vi "G#Template_CreateSub.vi"(0 "reference in":refnum<class "G#Template.lvclass">, 5 "error in (no error)":errorcluster) -> (14 "reference out":refnum<class "G#Template.lvclass">, 19 "error out":errorcluster)   [LabVIEW 2020, in "G#Template.lvclass"]
doc: "Constructor."
uses:
  G#Template.lvclass
  C:/ProjectGSharpDevelopment_2020-3/gsharp/VIPM/Files/vi.lib/addons/_AddQ/G#Object/G#Object.lvclass
  G#Object/G#Object.lvclass
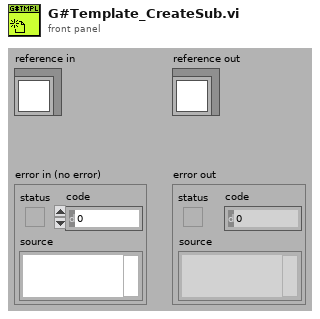
[diagram p1: front panel]
types:
  T1 = typedef "G#Template.lvclass/ObjectAttributesRef.ctl" = refnum<data-value>
  T2 = typedef "G#Template.lvclass/ObjectAttributes.ctl" = cluster{"MyAttribute":dbl}
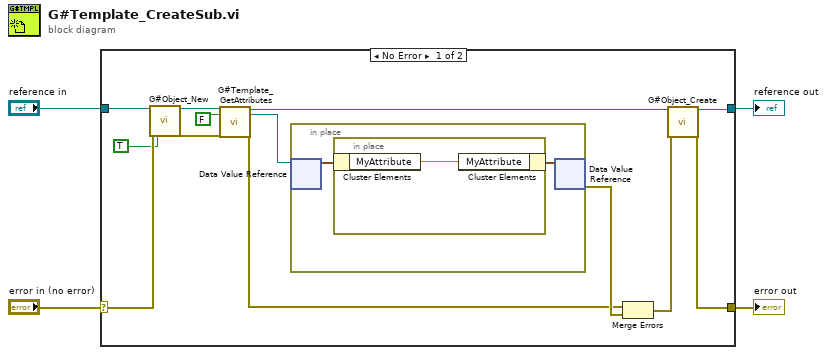
[diagram p0: block diagram]
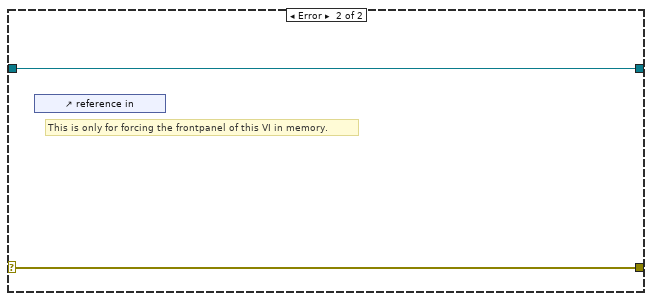
[diagram p2: hidden frame]
diagram:
  n1 = case shown="No Error" "error in (no error)" {
    selector: "error in (no error)" -> [w16 w22]
    tunnel: [w6 w22] -> w3
    tunnel: [w8 w21] -> w1
    tunnel: "reference in" -> [w17 w21]
    frame No Error {
      n2 = call "G#Object_New.vi"("reference in"=w17, "error in (no error)"=w16, "user counter (T)?"=TRUE ("User Counter")) -> ("reference out"=w11:refnum<class "G#Template.lvclass">, "error out"=w10:errorcluster)  [unwired: 14 in, 1 out]
      n3 = call "G#Template_GetAttributes.vi"("reference in"=w11, "return data? (T)"=FALSE ("return data"), "error in (no error)"=w10) -> ("reference out"=w9:refnum<class "G#Template.lvclass">, "attributes ref"=w13:T1, "error out"=w5:errorcluster)  [unwired: 13 in, 1 out]
      n4 = in-place {
        n5 = in-place-dvr #1(w13) -> (w18:T2)  [unwired: 1 out]
        n6 = in-place {
          n7 = in-place-cluster #2(w18) -> ("MyAttribute"=w20:dbl)
          n8 = in-place-cluster #2("MyAttribute"=w20) -> (w19:T2)
        }
        n9 = in-place-dvr #1(w19) -> (w14:errorcluster)  [unwired: 1 out]
      }
      n10 = Merge Errors(w5, w14) -> (w7:errorcluster)
      n11 = call-dynamic "G#Object_Create.vi"("reference in"=w9, "error in (no error)"=w7) -> ("reference out"=w8:refnum<class "G#Template.lvclass">, "error out"=w6:errorcluster)  [unwired: 16 in]
    }
    frame Error {
      # "This is only for forcing the frontpanel of this VI in memory."
      n12 = control-ref of="reference in"() -> ()  [unwired: 1 out]
    }
  }
  "error out" <- w3
  "reference out" <- w1
